vi "ManipAutoTarget.vi"(2 "Time Since Latch":u32, 3 "Instruction String":string) -> (0 "Error Out":errorcluster, 1 "Advance Trigger":bool)   [LabVIEW 2019]
doc: "This VI enters or exists auto-targeting mode.\n\nParameters:\n1. mode --> \"0\" exits auto-targeting while \"1\" enters auto-targeting"
uses:
  SafeParser_Integer.vi
  dsinstructions.vi
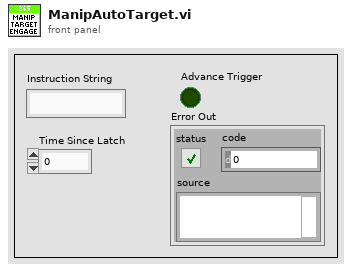
[diagram p1: front panel]
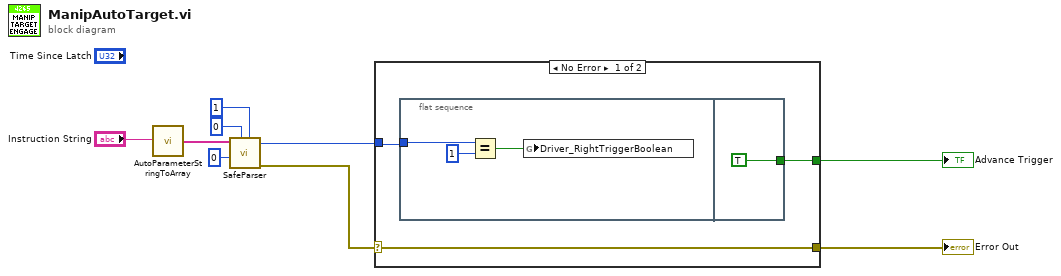
[diagram p0: block diagram]
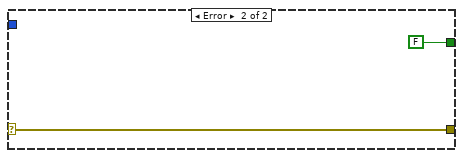
[diagram p2: hidden frame]
diagram:
  n1 = call "AutoParameterStringToArray.vi"("Parameter String"="Instruction String") -> ("Parsed Parameters"=w4:string[])
  n2 = call-poly "SafeParser.vi"("Maximum"=1, "Minimum"=0, "Array Index"=0 ("Parameter Index"), "String Array"=w4) -> ("Error Out"=w2:errorcluster, "Typecast  Value"=w3:i32)  [unwired: 6 in]
  n3 = case shown="No Error" w2 {
    selector: w2 -> [w11 w17]
    tunnel: [w12 FALSE ("Advance Trigger")] -> w9
    tunnel: [w11 w17] -> w8
    tunnel: w3 -> [w10 _]
    frame No Error {
      n4 = flat-sequence {
        tunnel: w10 -> [w15]
        tunnel: [TRUE ("Advance Trigger")] -> w12
        frame #0 {
          n5 = Equal?(x=w15, y=1) -> (x = y?=w13:bool)
          n6 = global write "dsinstructions.vi" "Driver_RightTriggerBoolean"(w13) -> ()
        }
        frame #1 {
        }
      }
    }
    frame Error {
    }
  }
  "Advance Trigger" <- w9
  "Error Out" <- w8
